vi "Configure AM Internal [AM] Core.vi"(7 "modulation waveform (Sine)":i32(ring)=1 items=["Sine"=1, "Square"=2, "Triangle"=3, "Ramp Up"=4, "Ramp Down"=5], 8 "error in (no error)":errorcluster, 9 "modulation frequency (1000 Hz)":dbl[unit]=1000.0 format="%^.2e", 10 "modulation depth (0.00 %)":dbl format="%.3f", 11 "IVI_Fgen in":refnum<class "IVI_Fgen.lvclass">) -> (0 "error out":errorcluster, 3 "IVI_Fgen out":refnum<class "IVI_Fgen.lvclass">)   [LabVIEW 2013, in "IVI_Fgen.lvlib" / "IVI_Fgen.lvclass"]
doc: "This VI configures the properties that control the function generator's internal amplitude modulation source. These properties are the modulation depth, waveform, and frequency.\n\nNotes:\n\n(1) This VI is part of the IviFgenModulateAM [AM] extension group."
uses:
  IVI_Fgen.lvclass
  IVI_Fgen.lvclass/IVI_Fgen.ctl
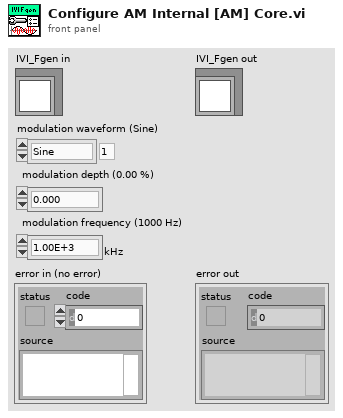
[diagram p1: front panel]
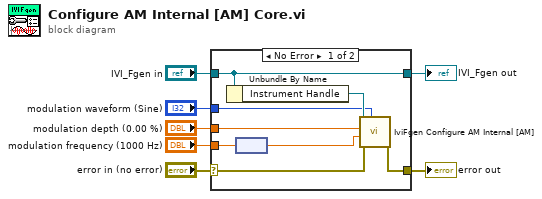
[diagram p0: block diagram]
diagram:
  n1 = case shown="No Error" "error in (no error)" {
    selector: "error in (no error)" -> [w13 w17]
    tunnel: [w12 w17] -> w6
    tunnel: [w15 w16] -> w4
    tunnel: "IVI_Fgen in" -> [w15 w16]
    tunnel: "modulation waveform (Sine)" -> [w11 _]
    tunnel: "modulation depth (0.00 %)" -> [w10 _]
    tunnel: "modulation frequency (1000 Hz)" -> [w9 _]
    frame No Error {
      n2 = Unbundle By Name(w15) -> ("Instrument Handle"=w14:refnum<k15>)
      n3 = node(w9) -> (w8:dbl)
      n4 = call <vilib>:"IviFgen Configure AM Internal [AM].vi"("modulation waveform (Sine)"=w11, "error in (no error)"=w13, "modulation frequency (1000 Hz)"=w8, "modulation depth (0.00 %)"=w10, "instrument handle"=w14) -> ("error out"=w12:errorcluster)  [unwired: 5 in, 1 out]
    }
    frame Error {
    }
  }
  "error out" <- w6
  "IVI_Fgen out" <- w4
